vi "hamamatsu_Read_functions.vi"() -> ()   [LabVIEW 2023]
panel:
  out "Function List":T1(array[cluster])
  out "error out":errorcluster
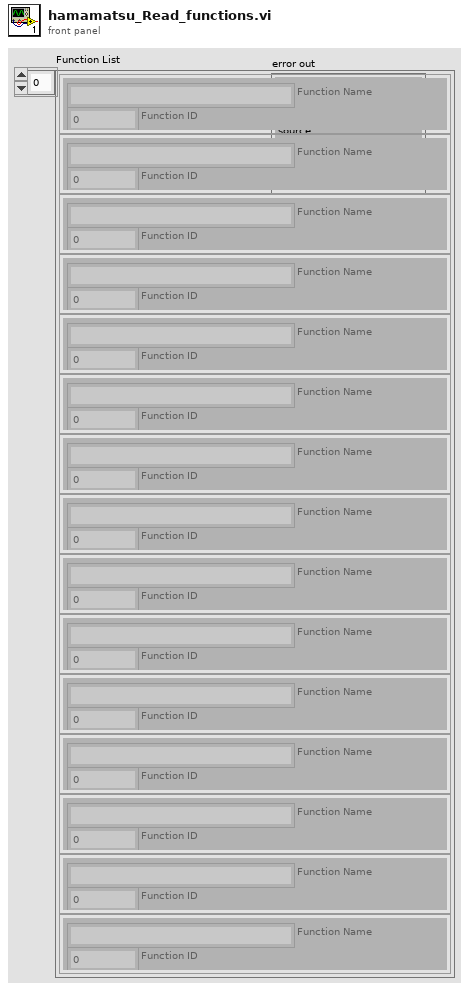
[diagram p1: front panel]
types:
  T1 = cluster{"Function Name":string, "Function ID":u32}[]
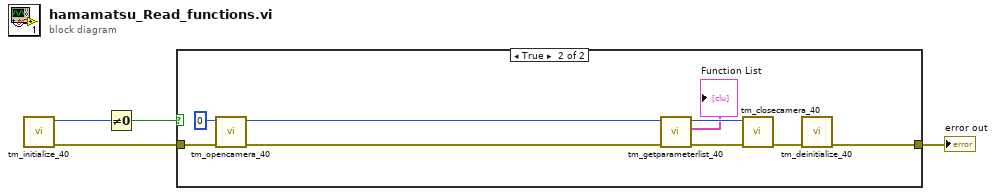
[diagram p0: block diagram]
diagram:
  n1 = call <userlib>:"tm_initialize_40.vi"() -> ("error out"=w3:errorcluster, "Number Of Cameras"=w4:u32)  [unwired: 8 in, 2 out]
  n2 = Not Equal To 0?(x=w4) -> (x != 0?=w2:bool)
  n3 = case shown="True" w2 {
    tunnel: w3 -> [w5 w14]
    tunnel: [w5 w9] -> w1
    frame False {
    }
    frame True {
      n4 = call <userlib>:"tm_opencamera_40.vi"("error in (no error)"=w14, "Camera Index"=u32 0) -> ("error out"=w12:errorcluster, "Handle out"=w11:u32)  [unwired: 7 in, 1 out]
      n5 = call <userlib>:"tm_getparameterlist_40.vi"("error in (no error)"=w12, "Handle in"=w11) -> ("error out"=w7:errorcluster, "Function List"=→"Function List":T1, "Handle out"=w8:u32)  [unwired: 7 in]
      n6 = call <userlib>:"tm_closecamera_40.vi"("error in (no error)"=w7, "Handle in"=w8) -> ("error out"=w10:errorcluster)  [unwired: 9 in]
      n7 = call <userlib>:"tm_deinitialize_40.vi"("error in (no error)"=w10) -> ("error out"=w9:errorcluster)  [unwired: 10 in]
    }
  }
  "error out" <- w1
